vi "Write Dev Elevator Config.vi"(8 "error in (no error)":errorcluster, 10 "Dev Elevator Config":T1, 11 "Dev Elevator in":refnum<class "Dev Elevator.lvclass">) -> (0 "error out":errorcluster, 3 "Dev Elevator out":refnum<class "Dev Elevator.lvclass">)   [LabVIEW 2014, in "Dev Elevator.lvlib" / "Dev Elevator.lvclass"]
uses:
  Dev Elevator.lvclass
  Dev Elevator Config.ctl
  <vilib>/Rock Robotics/WPI/Solenoid/WPI_SolenoidChannel.ctl
  Dev Elevator.lvclass/Dev Elevator.ctl
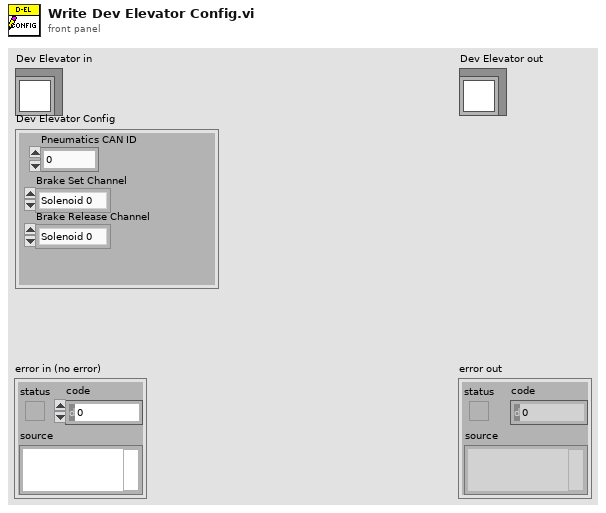
[diagram p1: front panel]
types:
  T1 = typedef "Dev Elevator.lvlib/Dev Elevator.lvclass/Dev Elevator Config.ctl" = cluster{"Brake Set Channel":T2, "Pneumatics CAN ID":u8, "Brake Release Channel":T2}
  T2 = typedef "WPI_SolenoidChannel.ctl" = enum8{"Solenoid 0", "Solenoid 1", "Solenoid 2", "Solenoid 3", "Solenoid 4", "Solenoid 5", "Solenoid 6", "Solenoid 7", "Invalid"}
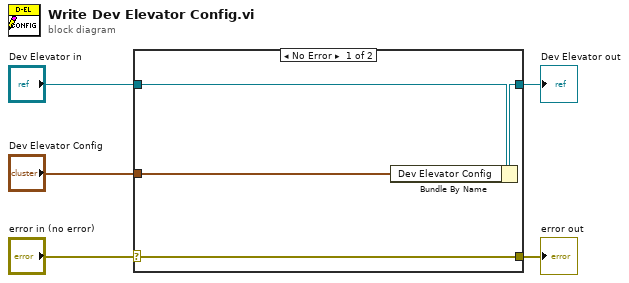
[diagram p0: block diagram]
diagram:
  n1 = case shown="No Error" "error in (no error)" {
    selector: "error in (no error)" -> [w9 w10]
    tunnel: [w9 w10] -> w4
    tunnel: [w7 w11] -> w2
    tunnel: "Dev Elevator in" -> [w8 w11]
    tunnel: "Dev Elevator Config" -> [w6 _]
    frame No Error {
      n2 = Bundle By Name(cluster=w8, "Dev Elevator Config"=w6) -> (w7:refnum<class "Dev Elevator.lvclass">)
    }
    frame Error {
    }
  }
  "error out" <- w4
  "Dev Elevator out" <- w2
